vi "Write MongoDB.Server.vi"(8 "error in (no error)":errorcluster, 10 "MongoDB.Server":refnum<k24>, 11 "MongoDB.Client in":refnum<class "MongoDB.Client.lvclass">) -> (0 "error out":errorcluster, 3 "MongoDB.Client out":refnum<class "MongoDB.Client.lvclass">)   [LabVIEW 2014, in "MongoDB.Client.lvclass"]
uses:
  MongoDB.Client.lvclass
  C:/MongoData/Drivers/mongo-csharp-driver-2.0.0-beta4/mongo-csharp-driver-2.0.0-beta4/src/MongoDB.Driver.Legacy/bin/Release/MongoDB.Driver.Legacy.dll
  MongoData/Drivers/mongo-csharp-driver-2.0.0-beta4/mongo-csharp-driver-2.0.0-beta4/src/MongoDB.Driver.Legacy/bin/Release/MongoDB.Driver.Legacy.dll
  MongoDB.Client.lvclass/MongoDB.Client.ctl
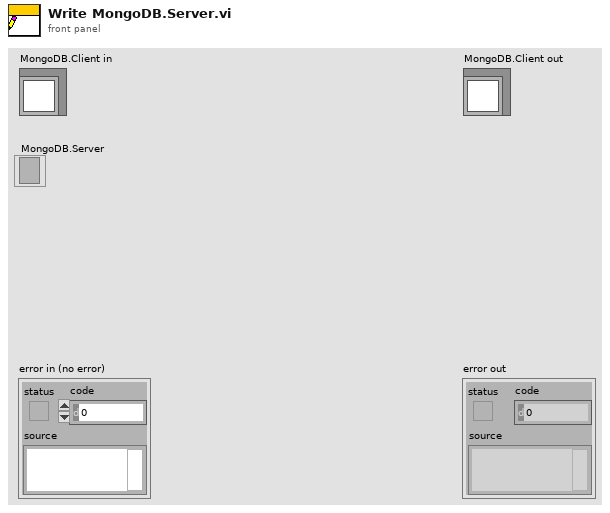
[diagram p1: front panel]
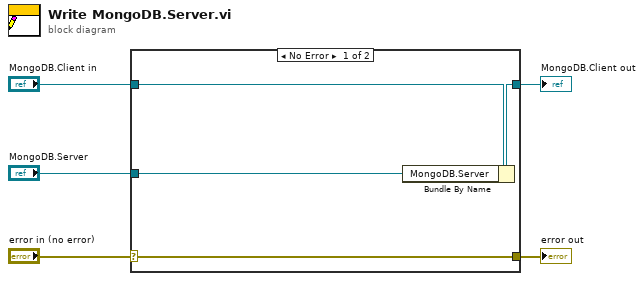
[diagram p0: block diagram]
diagram:
  n1 = case shown="No Error" "error in (no error)" {
    selector: "error in (no error)" -> [w9 w10]
    tunnel: [w9 w10] -> w4
    tunnel: [w7 w11] -> w2
    tunnel: "MongoDB.Client in" -> [w8 w11]
    tunnel: "MongoDB.Server" -> [w6 _]
    frame No Error {
      n2 = Bundle By Name(cluster=w8, "MongoDB.Server"=w6) -> (w7:refnum<class "MongoDB.Client.lvclass">)
    }
    frame Error {
    }
  }
  "error out" <- w4
  "MongoDB.Client out" <- w2
